vi "myRIO_BRig_RT__Case_Exp_State_SelectPre__v3.vi"(0 "input_dataCurrent":u16[](array[numeric]), 1 "input_SelectWrong":bool, 2 "input_SelectReward":bool, 5 "input_dataExp":u16[](array[numeric]), 11 "input_arrTrig":bool[](array[boolean])) -> (3 "output_state":T1, 4 "output_dataCurrent":u16[](array[numeric]), 8 "output_l1_laserEvent":bool, 10 "output_l1_laserOn":bool, 13 "output_l2_laserOn":bool, 14 "output_l2_laserEvent":bool)   [LabVIEW 2014]
uses:
  myRIO_BRig_RT__Case_Exp_stateList.ctl
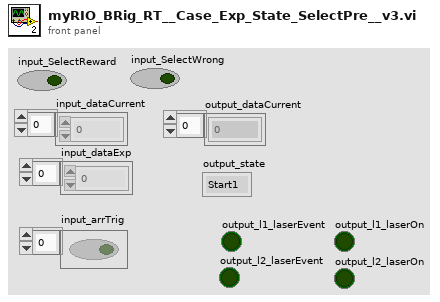
[diagram p1: front panel]
types:
  T1 = typedef "myRIO_BRig_RT__Case_Exp_stateList.ctl" = enum16{"Start1", "Start2", "Start3", "saveSettings1", "saveSettings2", "saveSettings3", "saveSettings4", "saveSettings_LC_ENL_l1", "saveSettings_LC_ENL_l2", "saveSettings_LC_Cue_l1", "saveSettings_LC_Cue_l2", "saveSettings6_LC_l1_Other", "SaveSettings6_LC_l2_Other", "setSettings_Audio", "setSettings_Laser", "initBlock_pre", "initBlock", "initBlock2", "initBlock_post", "initTrial_pre", "initTrial", "initTrial2", "initTrial3", "initTrial4", "initTrial_LC_ENL1", "initTrial_LC_Cue1", "initTrial_LC_Cue1_2", "initTrial_LC_Sel", "initTrial_post", "ENL1_pre", "ENL1", "ENL1_post", "ENL1Penalty_pre", "ENL1Penalty", "ENL2_pre", "ENL2", "ENL2Penalty_pre", "ENL2Penalty", "Cue1_pre", "Cue1", "Cue1_post", "Cue1Penalty_pre", "Cue1Penalty", "Cue2_pre", "Cue2", "Cue2Penalty_pre", "Cue2Penalty", "Selection_pre", "Selection", "Select_post", "SelectReward_pre", "SelectReward", "SelectRewardPost_pre", "SelectRewardPost", "SelectWrong_pre", "SelectWrong", "SelectWrong_post", "SelectTimeout_pre", "SelectTimeout", "SelectTimeout_post", "endTrial_pre", "endTrial1", "endTrial2", "endTrial3", "endTrial_post", "endBlock_pre", "endBlock", "endBlock_post", "endExp", "commConnect", "commUpload_pre", "commUpload_dataBlock", "commUpload_dataCurrent", "commUpload_dataExp", "commUpload_dataLC", "commUpload_dataTrial", "commUpload_post", "saveData_pre", "saveData_dataBlock", "saveData_dataCurrent", "saveData_dataExp", "saveData_dataLC", "saveData_dataTrial", "saveData_post", "empty_endBlock1", "empty_endBlock2", "empty_endTrial1", "empty_endTrial2", "empty_endTrial3", "empty_endTrial4", "empty_endTrial5", "dummyState", "dummyState_endBlock"}
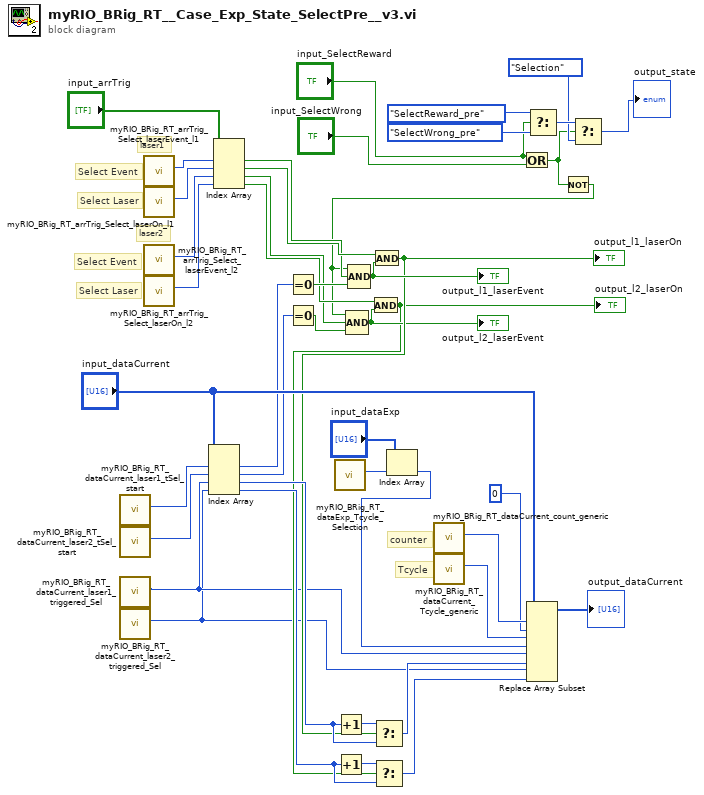
[diagram p0: block diagram]
diagram:
  # "Select Event"
  # "Select Laser"
  # "Select Event"
  # "Select Laser"
  # "laser2"
  # "laser1"
  # "Tcycle"
  # "counter"
  n1 = call "myRIO_BRig_RT_dataCurrent_laser1_tSel_start.vi"() -> ("output_laser1_tSel_start"=w11:i32)  [unwired: 11 in]
  n2 = call "myRIO_BRig_RT_dataCurrent_laser2_tSel_start.vi"() -> ("output_laser2_tSel_start"=w12:i32)  [unwired: 11 in]
  n3 = call "myRIO_BRig_RT_dataCurrent_laser1_triggered_Sel.vi"() -> ("output_laser1_triggered_Selection"=w8:i32)  [unwired: 11 in]
  n4 = call "myRIO_BRig_RT_dataCurrent_laser2_triggered_Sel.vi"() -> ("output_laser2_triggered_Selection"=w7:i32)  [unwired: 11 in]
  n5 = call "myRIO_BRig_RT_arrTrig_Select_laserEvent_l1.vi"() -> ("output_arrTrig_Select_laserEvent_l1"=w27:i32)  [unwired: 11 in]
  n6 = call "myRIO_BRig_RT_arrTrig_Select_laserOn_l1.vi"() -> ("output_arrTrig_Select_laserOn_l1"=w26:i32)  [unwired: 11 in]
  n7 = call "myRIO_BRig_RT_arrTrig_Select_laserEvent_l2.vi"() -> ("output_arrTrig_Select_laserEvent_l2"=w25:i32)  [unwired: 11 in]
  n8 = call "myRIO_BRig_RT_arrTrig_Select_laserOn_l2.vi"() -> ("output_arrTrig_Select_laserOn_l2"=w24:i32)  [unwired: 11 in]
  n9 = Index Array(array="input_dataCurrent", index #1=w11, index #2=w12, index #3=w8, index #4=w7) -> (element #1=w40:u16, element #2=w39:u16, element #3=w36:u16, element #4=w35:u16)
  n10 = Index Array(array="input_arrTrig", index #1=w27, index #2=w26, index #3=w25, index #4=w24) -> (element #1=w19:bool, element #2=w20:bool, element #3=w21:bool, element #4=w22:bool)
  n11 = Equal To 0?(x=w40) -> (x = 0?=w34:bool)
  n12 = Equal To 0?(x=w39) -> (x = 0?=w29:bool)
  n13 = call "myRIO_BRig_RT_dataExp_Tcycle_Selection.vi"() -> ("output_Tcycle_Selection"=w2:i32)  [unwired: 11 in]
  n14 = Increment(x=w36) -> (x+1=w38:u16)
  n15 = Increment(x=w35) -> (x+1=w37:u16)
  n16 = Index Array(array="input_dataExp", index=w2) -> (element=w1:u16)
  n17 = call "myRIO_BRig_RT_dataCurrent_count_generic.vi"() -> ("output_count_generic"=w43:i32)  [unwired: 11 in]
  n18 = call "myRIO_BRig_RT_dataCurrent_Tcycle_generic.vi"() -> ("output_Tcycle_generic"=w42:i32)  [unwired: 11 in]
  n19 = Or(x="input_SelectReward", y="input_SelectWrong") -> (x .or. y?=w6:bool)
  n20 = Select(t=myRIO_BRig_RT__Case_Exp_stateList."SelectReward_pre" ("Enum"), s="input_SelectReward", f=myRIO_BRig_RT__Case_Exp_stateList."SelectWrong_pre" ("Enum")) -> (s? t:f=w18:T1)
  n21 = Not(x=w6) -> (.not. x?=w5:bool)
  n22 = Compound Arithmetic op=AND(w5, w21, w29) -> (w31:bool)
  "output_l2_laserEvent" <- w31
  n23 = Compound Arithmetic op=AND(w5, w19, w34) -> (w33:bool)
  "output_l1_laserEvent" <- w33
  n24 = And(x=w22, y=w31) -> (x .and. y?=w30:bool)
  "output_l2_laserOn" <- w30
  n25 = And(x=w20, y=w33) -> (x .and. y?=w32:bool)
  "output_l1_laserOn" <- w32
  n26 = Select(t=w38, s=w32, f=w36) -> (s? t:f=w10:u16)
  n27 = Select(t=w37, s=w30, f=w35) -> (s? t:f=w9:u16)
  n28 = Replace Array Subset(array="input_dataCurrent", new element #1=u16 0 ("new element/subarray"), index #1=w43, new element #2=w1, index #2=w42, new element #3=w10, index #3=w8, new element #4=w9, index #4=w7) -> (→"output_dataCurrent":u16[])
  n29 = Select(t=w18, s=w6, f=myRIO_BRig_RT__Case_Exp_stateList."Selection" ("Enum")) -> (s? t:f=→"output_state":T1)
